vi "set pockels cell.vi"(8 "error in (no error)":errorcluster, 11 "ImagingModeSPIM in":refnum<class "ImagingModeSPIM.lvclass">) -> (0 "error out":errorcluster, 3 "ImagingModeSPIM out":refnum<class "ImagingModeSPIM.lvclass">)   [LabVIEW 2012, in "ImagingModeSPIM.lvclass"]
uses:
  ImagingModeSPIM.lvclass
  ImagingModeSPIM.lvclass/ImagingModeSPIM.ctl
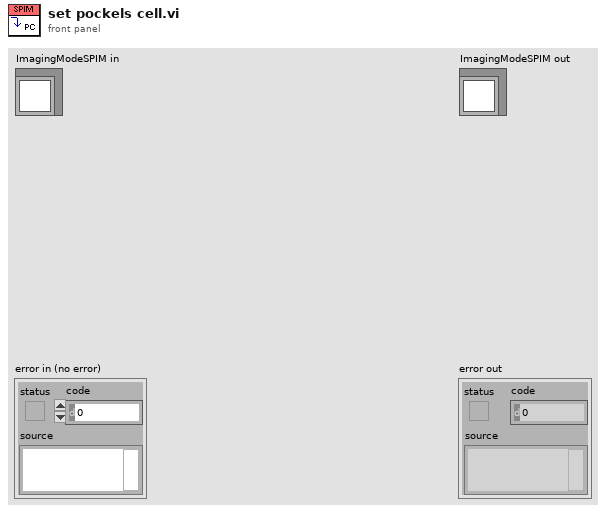
[diagram p1: front panel]
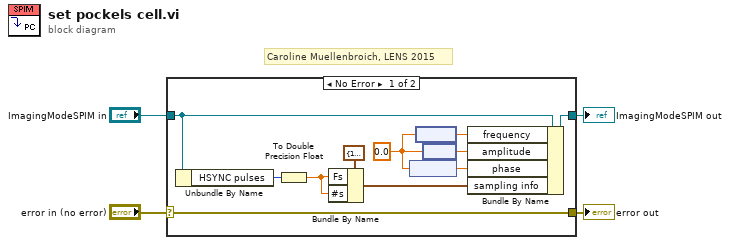
[diagram p0: block diagram]
diagram:
  # "Caroline Muellenbroich, LENS 2015"
  n1 = case shown="No Error" "error in (no error)" {
    selector: "error in (no error)" -> [w15 w17]
    tunnel: [w15 w17] -> w3
    tunnel: [w14 w16] -> w1
    tunnel: "ImagingModeSPIM in" -> [w9 w16]
    frame No Error {
      w13 = 0.0 ("settings.Pockels Cell.frequency")
      n2 = Unbundle By Name(w9) -> ("HSYNC pulses"=w6:i32)
      n3 = To Double Precision Float(number=w6) -> (double precision float=w8:dbl)
      n4 = Bundle By Name(cluster=cluster{"Fs":dbl, "#s":dbl} {"Fs"=1000.0, "#s"=1000.0} ("sampling info 2"), "Fs"=w8, "#s"=w8) -> (w5:cluster{"Fs":dbl, "#s":dbl})
      n5 = node(w13) -> (w12:dbl[unit])
      n6 = node(w13) -> (w10:dbl[unit])
      n7 = node(w13) -> (w11:dbl[unit])
      n8 = Bundle By Name(cluster=w9, "frequency"=w10, "amplitude"=w11, "phase"=w12, "sampling info"=w5) -> (w14:refnum<class "ImagingModeSPIM.lvclass">)
    }
    frame Error {
    }
  }
  "error out" <- w3
  "ImagingModeSPIM out" <- w1
